vi "oneButtonNotify.vi"(2 "message":string) -> (0 "stop":bool)   [LabVIEW 2024]
panel:
  in  "Boolean":bool
  out "message":string
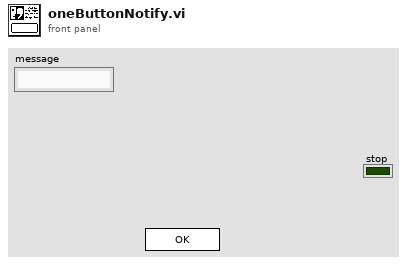
[diagram p1: front panel]
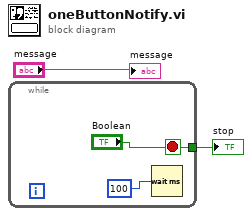
[diagram p0: block diagram]
diagram:
  n1 = while {
    tunnel: ["Boolean"] -> w1
    stop <- "Boolean" stop-if-true
    n2 = Wait (ms)(milliseconds to wait=u32 100 ("millisecond timer value")) -> ()  [unwired: 1 out]
  }
  "stop" <- w1
  "message" <- "message"
